vi "总磷总氮MB_api.vi"(6 "Slave ID":u8=1, 7 "STEP":enum16{"open", "read", "write", "close"}(ring)=enum."read", 8 "Error in":errorcluster caption="Error in (no error)", 9 "values":u16[](array[numeric]), 10 "quantity":u16, 11 "starting address":u16 format="%04xH") -> (0 "error out":errorcluster, 2 "MB session out":refnum<class "MB_Master.lvclass">, 3 "Registers":u16[](array[numeric]))   [LabVIEW 2016, in "斯坦道通用流路CODmn.lvlib"]
uses:
  <vilib>/Plasmionique/MB Master/MB_Master/MB_Master.lvclass
  <vilib>/Plasmionique/MB Master/MB_Master_Serial/MB_Master_Serial.lvclass
  C:/Program Files (x86)/National Instruments/LabVIEW 2016/vi.lib/Plasmionique/MB Master/MB_Master/MB_Master.lvclass
  <vilib>/Plasmionique/MB Master/MB_Master_TCP/MB_Master_TCP.lvclass
  <vilib>/Plasmionique/MB Master/MB Master.lvlib
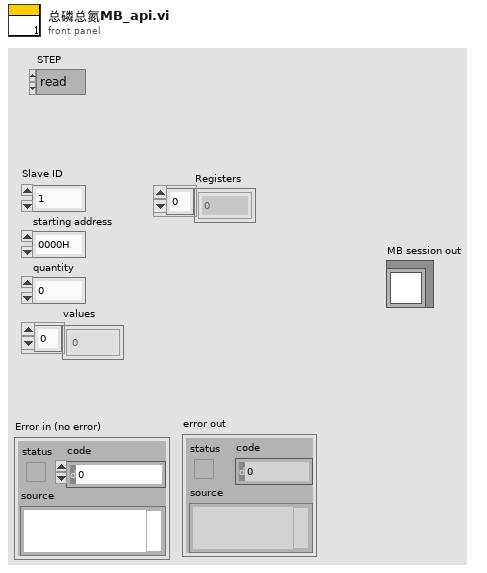
[diagram p1: front panel]
types:
  T1 = cluster{"baud rate (bps)":u32, "stop bits":u16, "parity":u16, "flow control":u16, "timeout":u32, "retries":i32}
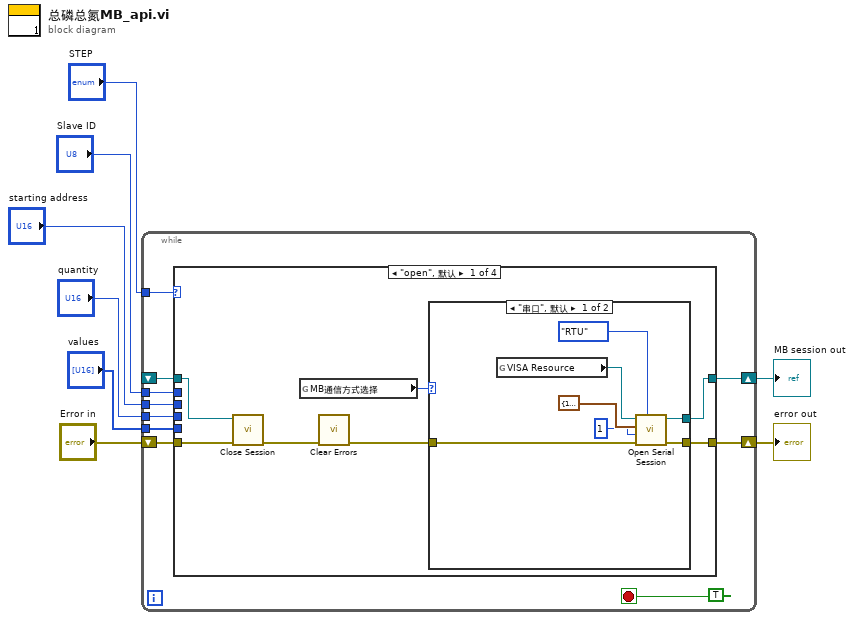
[diagram p0: block diagram]
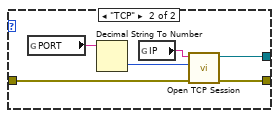
[diagram p2: hidden frame]
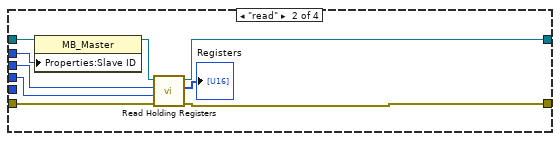
[diagram p3: hidden frame]
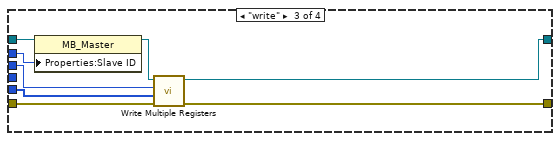
[diagram p4: hidden frame]
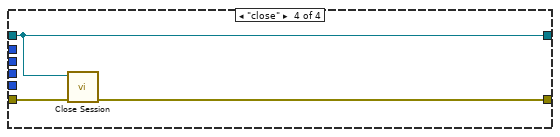
[diagram p5: hidden frame]
diagram:
  n1 = while {
    shift-right: [w9] -> w1
    shift-left: _ -> [w18]
    shift-right: [w10] -> w7
    shift-left: "Error in" -> [w17]
    tunnel: "Slave ID" -> [w16]
    tunnel: "starting address" -> [w15]
    tunnel: "quantity" -> [w14]
    tunnel: "STEP" -> [w13]
    tunnel: "values" -> [w12]
    stop <- TRUE stop-if-true
    n2 = case shown="\"open\", 默认" w13 {
      tunnel: w18 -> [w24 w40 w53 w56]
      tunnel: w17 -> [w23 w47 w55 w58]
      tunnel: [w19 w46 w52 w56] -> w9
      tunnel: [w25 w45 w54 w57] -> w10
      tunnel: w16 -> [_ w43 w48 _]
      tunnel: w15 -> [_ w42 w51 _]
      tunnel: w14 -> [_ w41 _ _]
      tunnel: w12 -> [_ _ w50 _]
      frame "open", Default {
        n3 = call-dynamic "Close Session.vi"("error in (no error)"=w23, "MB session in"=w24) -> ("error out"=w21:errorcluster)  [unwired: 9 in]
        n4 = global read "总磷总氮断电保存全局变量.vi" "MB通信方式选择"() -> (w22:enum16{"串口", "TCP"})
        n5 = call <vilib>:"Clear Errors.vi"("error in (no error)"=w21) -> ("error out"=w20:errorcluster)  [unwired: 5 in, 1 out]
        n6 = case shown="\"串口\", 默认" w22 {
          tunnel: [w30 w36] -> w25
          tunnel: [w26 w35] -> w19
          tunnel: w20 -> [w28 w37]
          frame "串口", Default {
            n7 = global read "总磷总氮断电保存全局变量.vi" "VISA Resource"() -> (w27:refnum<visa-resource-name>)
            n8 = call <vilib>:"Open Serial Session.vi"("Mode (RTU)"=enum16{"RTU", "ASCII"}."RTU", "Error in"=w28, "Slave ID"=u8 1, "Serial Config"=T1 {"baud rate (bps)"=115200, "stop bits"=10, "parity"=0, "flow control"=0, "timeout"=1000, "retries"=1}, "VISA Resource"=w27) -> ("Error out"=w30:errorcluster, "MB_Serial session"=w26:refnum<class "MB_Master_Serial.lvclass">)  [unwired: 5 in]
          }
          frame "TCP" {
            n9 = global read "总磷总氮断电保存全局变量.vi" "PORT"() -> (w34:string)
            n10 = Decimal String To Number(string=w34) -> (number=w38:i32)  [unwired: 2 in, 1 out]
            n11 = global read "总磷总氮断电保存全局变量.vi" "IP"() -> (w33:string)
            n12 = call <vilib>:"Open TCP Session.vi"("error in (no error)"=w37, "Port (502)"=w38, "IP Address"=w33) -> ("error out"=w36:errorcluster, "MB_TCP session"=w35:refnum<class "MB_Master_TCP.lvclass">)  [unwired: 7 in]
          }
        }
      }
      frame "read" {
        n13 = property class="MB_Master"(reference=w40, "Properties:Slave ID"=w43) -> (reference out=w39:refnum<class "MB_Master.lvclass">)  [unwired: 1 in, 1 out]
        n14 = call <vilib>:"Read Holding Registers.vi"("error in (no error)"=w47, "quantity"=w41, "starting address"=w42, "MB session in"=w39) -> ("error out"=w45:errorcluster, "Registers"=→"Registers":u16[], "MB session out"=w46:refnum<class "MB_Master.lvclass">)  [unwired: 5 in]
      }
      frame "write" {
        n15 = property class="MB_Master"(reference=w53, "Properties:Slave ID"=w48) -> (reference out=w49:refnum<class "MB_Master.lvclass">)  [unwired: 1 in, 1 out]
        n16 = call <vilib>:"Write Multiple Registers.vi"("error in (no error)"=w55, "values"=w50, "starting address"=w51, "MB session in"=w49) -> ("error out"=w54:errorcluster, "MB session out"=w52:refnum<class "MB_Master.lvclass">)  [unwired: 6 in]
      }
      frame "close" {
        n17 = call-dynamic "Close Session.vi"("error in (no error)"=w58, "MB session in"=w56) -> ("error out"=w57:errorcluster)  [unwired: 9 in]
      }
    }
  }
  "error out" <- w7
  "MB session out" <- w1
